vi "Read Known Host Data.vi"(8 "error in (no error)":errorcluster, 11 "known host":T1) -> (0 "error out":errorcluster, 2 "known host data":T2)   [LabVIEW 2013, in "libssh2.lvlib"]
doc: "Reads information from <B>known host</B>."
uses:
  libssh2.lvlib
  libssh2_knownhost.ctl
  Known Host Refnum.ctl
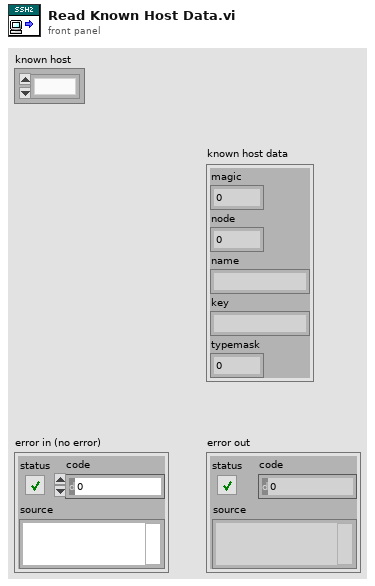
[diagram p1: front panel]
types:
  T1 = typedef "libssh2.lvlib/Known Host Refnum.ctl" = refnum<k1>
  T2 = typedef "libssh2.lvlib/libssh2_knownhost.ctl" = cluster{"magic":u32, "node":u64, "name":string, "key":string, "typemask":i32}
  T3 = cluster{"magic":u32, "node":u64, "name":u64, "key":u64, "typemask":i32}
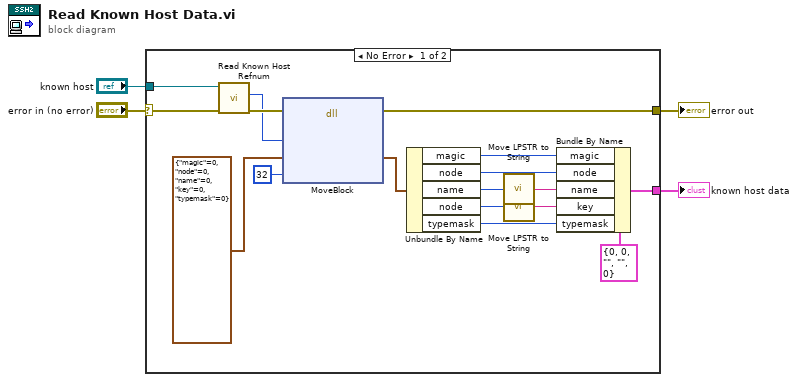
[diagram p0: block diagram]
diagram:
  n1 = case shown="No Error" "error in (no error)" {
    selector: "error in (no error)" -> [w5 w22]
    tunnel: [w21 _] -> w4
    tunnel: "known host" -> [w18 _]
    tunnel: [w17 w22] -> w2
    frame No Error {
      n2 = call "Read Known Host Refnum.vi"("error in (no error)"=w5, "known host"=w18) -> ("error out"=w19:errorcluster, "libssh2_knownhost*"=w16:u64)  [unwired: 8 in]
      n3 = dll-call lib="LabVIEW" fn="MoveBlock"(error in=w19, "ps"=w16, T3 {"magic"=0, "node"=0, "name"=0, "key"=0, "typemask"=0}, "size"=i64 32) -> (error out=w17:errorcluster, w13:T3)  [unwired: 5 in, 1 out]
      n4 = Unbundle By Name(w13) -> ("magic"=w11:u32, "node"=w10:u64, "name"=w12:u64, "node"=w8:u64, "typemask"=w6:i32)
      n5 = call "Move LPSTR to String.vi"("LPSTR"=w12) -> ("String"=w9:string)  [unwired: 1 in]
      n6 = call "Move LPSTR to String.vi"("LPSTR"=w8) -> ("String"=w7:string)  [unwired: 1 in]
      n7 = Bundle By Name(cluster=T2 {"magic"=0, "node"=0, "name"="", "key"="", "typemask"=0} ("libssh2_knownhost"), "magic"=w11, "node"=w10, "name"=w9, "key"=w7, "typemask"=w6) -> (w21:T2)
    }
    frame Error {
    }
  }
  "known host data" <- w4
  "error out" <- w2
